vi "Init.vi"(0 "object in":refnum<class "ExtraGUI.lvclass">, 1 "IniFile":path, 5 "error in (no error)":errorcluster) -> (14 "object out":refnum<class "ExtraGUI.lvclass">, 19 "error out":errorcluster)   [LabVIEW 2017, in "ExtraGUI.lvclass"]
uses:
  ExtraGUI.lvclass
  ExtraGUI.lvclass/ExtraGUI.ctl
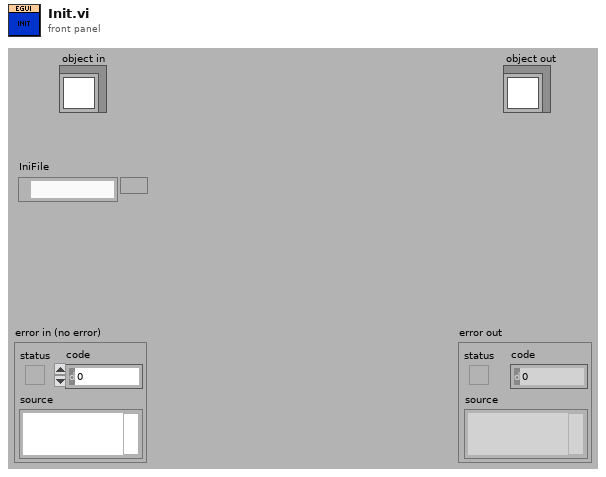
[diagram p1: front panel]
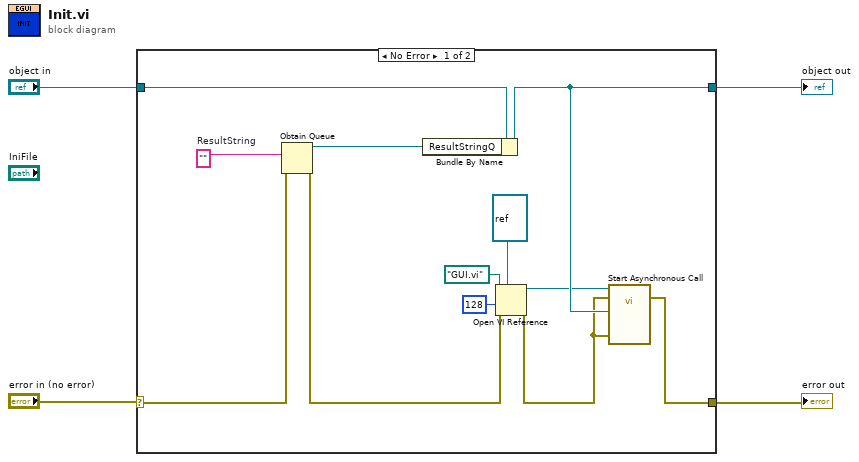
[diagram p0: block diagram]
diagram:
  n1 = case shown="No Error" "error in (no error)" {
    selector: "error in (no error)" -> [w13 w17]
    tunnel: "object in" -> [w16 w18]
    tunnel: [w9 w18] -> w3
    tunnel: [w6 w17] -> w1
    frame No Error {
      w15 = ""  # ResultString
      n2 = Obtain Queue(element data type=w15, error in (no error)=w13) -> (queue out=w14:refnum<queue>, error out=w7:errorcluster)  [unwired: 3 in, 1 out]
      n3 = Bundle By Name(cluster=w16, "ResultStringQ"=w14) -> (w9:refnum<class "ExtraGUI.lvclass">)
      n4 = Open VI Reference(type specifier VI Refnum (for type only)=refnum<vi> refnum, vi path=path "GUI.vi", options=128, error in (no error)=w7) -> (vi reference=w8:refnum<vi>, error out=w5:errorcluster)  [unwired: 1 in, 1 out]
      n5 = call-by-ref "Start Asynchronous Call"(reference=w8, error in=w5, 8:"error in (no error)"=w5, "object in"=w9) -> (error out=w6:errorcluster)  [unwired: 8 in, 3 out]
    }
    frame Error {
    }
  }
  "object out" <- w3
  "error out" <- w1
